vi "Distance.vi"(8 "y2":dbl, 9 "y1":dbl, 10 "x2":dbl, 11 "x1":dbl) -> (3 "Dist":dbl)   [LabVIEW 2011]
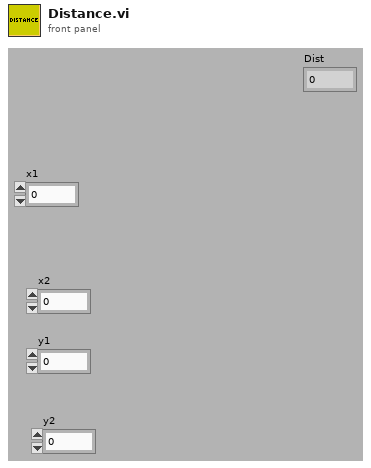
[diagram p1: front panel]
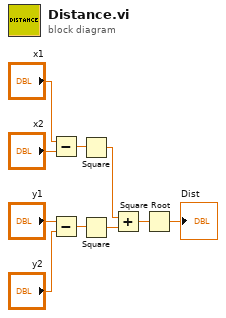
[diagram p0: block diagram]
diagram:
  n1 = Subtract(x="x1", y="x2") -> (x-y=w6:dbl)
  n2 = Subtract(x="y1", y="y2") -> (x-y=w5:dbl)
  n3 = Square(x=w6) -> (x^2=w4:dbl)
  n4 = Square(x=w5) -> (x^2=w3:dbl)
  n5 = Add(x=w4, y=w3) -> (x+y=w2:dbl)
  n6 = Square Root(x=w2) -> (sqrt(x)=→"Dist":dbl)
